vi "Get Entry.vi"(8 "error in":errorcluster, 11 "Object Entry in":refnum<class "Object Entry.lvclass">) -> (0 "error out":errorcluster, 3 "Object Entry out":refnum<class "Object Entry.lvclass">)   [LabVIEW 2024, in "EDS.lvlib" / "Object Entry.lvclass"]
uses:
  Object Entry.lvclass
  Object Entry.lvclass/Object Entry.ctl
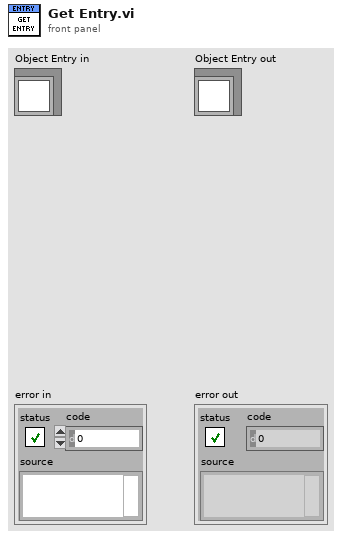
[diagram p1: front panel]
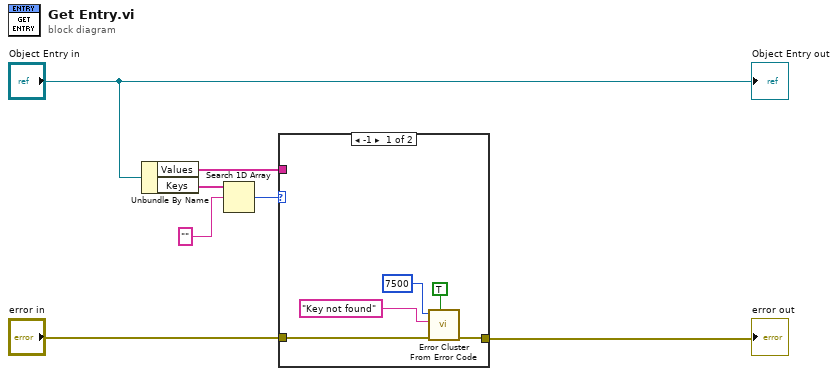
[diagram p0: block diagram]
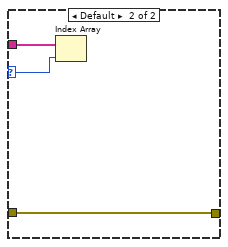
[diagram p2: hidden frame]
diagram:
  n1 = Unbundle By Name("Object Entry in") -> ("Values"=w2:string[], "Keys"=w6:string[])
  n2 = Search 1D Array(1D array=w6, element="") -> (index of element=w5:i32)  [unwired: 1 in]
  n3 = case shown="-1" w5 {
    selector: w5 -> [_ w14]
    tunnel: "error in" -> [w12 w13]
    tunnel: [w8 w13] -> w3
    tunnel: w2 -> [_ w15]
    frame -1 {
      n4 = call <vilib>:"Error Cluster From Error Code.vi"("show call chain? (False)"=TRUE, "error in (no error)"=w12, "error message (\"\")"="Key not found" ("error message (\"\")"), "error code (0)"=7500) -> ("error out"=w8:errorcluster)  [unwired: 5 in]
    }
    frame Default {
      n5 = Index Array(array=w15, index=w14) -> ()  [unwired: 1 out]
    }
  }
  "error out" <- w3
  "Object Entry out" <- "Object Entry in"
